vi "Init Menu.vi"(8 "Error In":errorcluster, 9 "Used Items":bool[](array[boolean]), 10 "Item Names":string[][](array[string]), 11 "Menu in":refnum<k9>) -> (0 "Error Out":errorcluster, 3 "menu reference out":refnum<k9>)   [LabVIEW 2019]
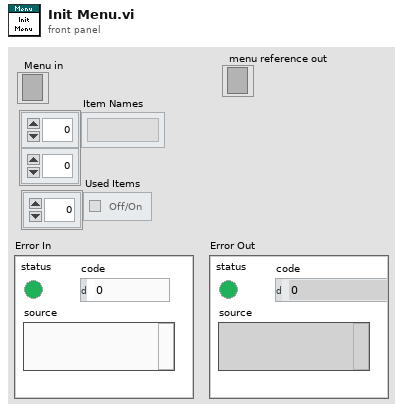
[diagram p1: front panel]
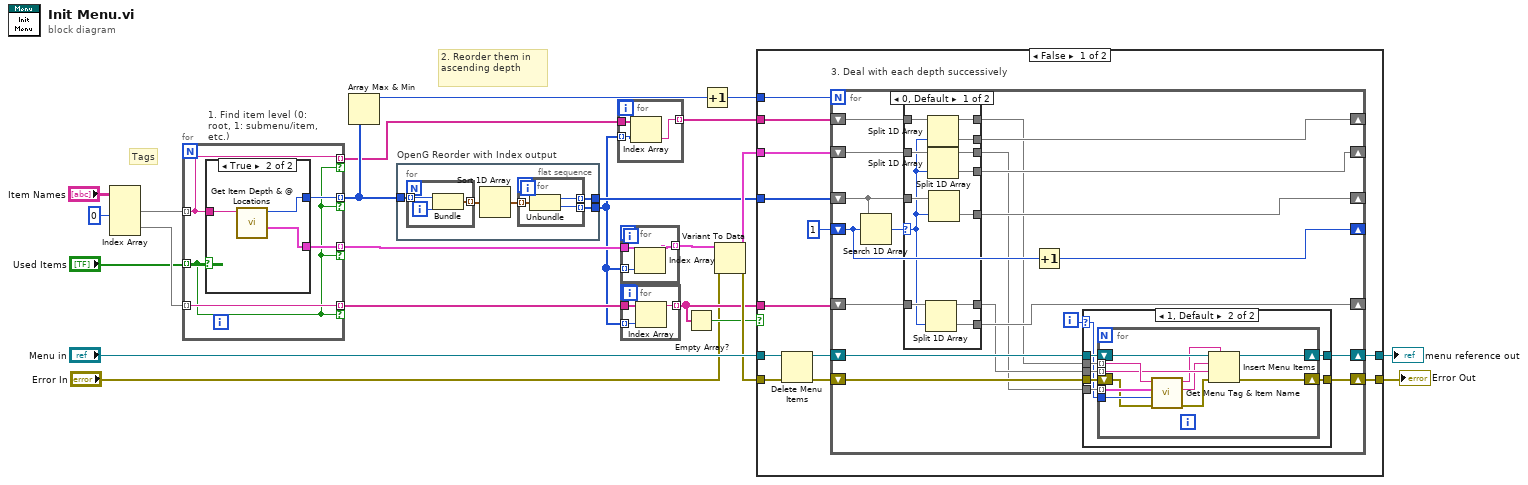
[diagram p0: block diagram]
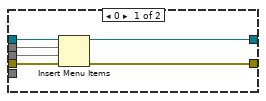
[diagram p3: hidden frame]
diagram:
  # "Tags"
  # "2. Reorder them in ascending depth"
  n1 = Index Array(array="Item Names", index (col) #1=0 ("disabled index (col)")) -> (element #1=w10:string[], element #2=w12:string[])  [unwired: 3 in]
  n2 = for "1. Find item level (0: root, 1: submenu/item, etc.)" {
    tunnel: w10 -> [w25] mode=indexing
    tunnel: [w28] -> w18 mode=indexing if=w24
    tunnel: [w27] -> w21 mode=indexing if=w24
    tunnel: "Used Items" -> [w24] mode=indexing
    tunnel: w12 -> [w26] mode=indexing
    tunnel: [w26] -> w11 mode=indexing if=w24
    tunnel: [w25] -> w1 mode=indexing if=w24
    n3 = case shown="True" w24 {
      tunnel: w25 -> [_ w31]
      tunnel: [_ w29] -> w28
      tunnel: [_ w30] -> w27
      frame False {
      }
      frame True {
        n4 = call "Get Item Depth & @ Locations.vi"("Menu Item Description"=w31) -> ("@ Locations"=w29:cluster{"Array":i32[]}, "Depth"=w30:i32)  [unwired: 8 in, 1 out]
      }
    }
  }
  n5 = Array Max & Min(array=w21) -> (max value=w20:i32)  [unwired: 3 out]
  n6 = flat-sequence "OpenG Reorder with Index output" {
    tunnel: w21 -> [w36]
    tunnel: [w35] -> w14
    tunnel: [w34] -> w3
    frame #0 {
      n7 = for {
        tunnel: w36 -> [w39] mode=indexing
        tunnel: [w37] -> w33 mode=indexing
        i -> [w38]
        n8 = Bundle("Depth"=w39, w38) -> (w37:cluster{"Depth":i32, i32})  [unwired: 1 in]
      }
      n9 = Sort 1D Array(array=w33) -> (sorted array=w32:cluster{"Depth":i32, i32}[])
      n10 = for {
        tunnel: w32 -> [w42] mode=indexing
        tunnel: [w40] -> w35 mode=indexing
        tunnel: [w41] -> w34 mode=indexing
        n11 = Unbundle(w42) -> ("Depth"=w40:i32, w41:i32)
      }
    }
  }
  n12 = for {
    tunnel: w1 -> [w45]
    tunnel: [w44] -> w16 mode=indexing
    tunnel: w3 -> [w43] mode=indexing
    n13 = Index Array(array=w45, index=w43) -> (element=w44:string)
  }
  n14 = for {
    tunnel: w18 -> [w48]
    tunnel: [w47] -> w19 mode=indexing
    tunnel: w3 -> [w46] mode=indexing
    n15 = Index Array(array=w48, index=w46) -> (element=w47:cluster{"Array":i32[]})
  }
  n16 = for {
    tunnel: w11 -> [w51]
    tunnel: [w50] -> w6 mode=indexing
    tunnel: w3 -> [w49] mode=indexing
    n17 = Index Array(array=w51, index=w49) -> (element=w50:string)
  }
  n18 = Empty Array?(array=w6) -> (empty?=w5:bool)
  n19 = Increment(x=w20) -> (x+1=w13:i32)
  n20 = Variant To Data(error in="Error In", type=w18, Variant=w19) -> (data=w17:cluster{"Array":i32[]}[], error out=w7:errorcluster)
  n21 = case shown="False" w5 {
    tunnel: "Menu in" -> [w63 w123]
    tunnel: w17 -> [w61 _]
    tunnel: w16 -> [w59 _]
    tunnel: [w58 w124] -> w15
    tunnel: w14 -> [w57 _]
    tunnel: w13 -> [w56 _]
    tunnel: w7 -> [w55 w124]
    tunnel: w6 -> [w53 _]
    tunnel: [w52 w123] -> w2
    frame False {
      n22 = Delete Menu Items(6:w55, 9:w63) -> (0:w54:errorcluster, 3:w60:refnum<k9>)  [unwired: 2 in]
      n23 = for "3. Deal with each depth successively" {
        N: w56 -> [_]
        shift-right: [w81] -> _
        shift-left: w57 -> [w82]
        shift-right: [w79] -> _
        shift-left: 1 ("max value") -> [w80]
        shift-right: [w77] -> _
        shift-left: w61 -> [w78]
        shift-right: [w75] -> _
        shift-left: w53 -> [w76]
        shift-right: [w73] -> w52
        shift-left: w60 -> [w74]
        shift-right: [w71] -> w58
        shift-left: w54 -> [w72]
        shift-right: [w67] -> _
        shift-left: w59 -> [w69]
        i -> [w65]
        n24 = Search 1D Array(1D array=w82, element=w80) -> (index of element=w68:i32)  [unwired: 1 in]
        n25 = case shown="0, Default" w68 {
          selector: w68 -> [w83 _]
          tunnel: w82 -> [w94 _]
          tunnel: [w93 _] -> w81
          tunnel: w78 -> [w92 w96]
          tunnel: [w91 _] -> w77
          tunnel: w76 -> [w90 w95]
          tunnel: [w89 _] -> w75
          tunnel: [w88 w95] -> w70
          tunnel: w69 -> [w87 w97]
          tunnel: [w86 _] -> w67
          tunnel: [w85 w97] -> w66
          tunnel: [w84 w96] -> w64
          frame 0, Default {
            n26 = Split 1D Array(array=w90, index=w83) -> (first subarray=w88:string[], second subarray=w89:string[])
            n27 = Split 1D Array(array=w87, index=w83) -> (first subarray=w85:string[], second subarray=w86:string[])
            n28 = Split 1D Array(array=w92, index=w83) -> (first subarray=w84:cluster{"Array":i32[]}[], second subarray=w91:cluster{"Array":i32[]}[])
            n29 = Split 1D Array(array=w94, index=w83) -> (second subarray=w93:i32[])  [unwired: 1 out]
          }
          frame -1 {
          }
        }
        n30 = Increment(x=w80) -> (x+1=w79:i32)
        n31 = case shown="1, Default" w65 {
          selector: w65 -> [_ w104]
          tunnel: w74 -> [w103 w111]
          tunnel: [w102 w110] -> w73
          tunnel: w72 -> [w101 w109]
          tunnel: [w99 w108] -> w71
          tunnel: w70 -> [w100 w106]
          tunnel: w66 -> [w98 w107]
          tunnel: w64 -> [_ w105]
          frame 0 {
            n32 = Insert Menu Items(6:w101, 7:w100, 8:w98, 9:w103) -> (0:w99:errorcluster, 3:w102:refnum<k9>)  [unwired: 2 in, 1 out]
          }
          frame 1, Default {
            n33 = for {
              shift-right: [w121] -> w110
              shift-left: w111 -> [w122]
              shift-right: [w114] -> w108
              shift-left: w109 -> [w116]
              tunnel: w107 -> [w120] mode=indexing
              tunnel: w106 -> [w119] mode=indexing
              tunnel: w105 -> [w118] mode=indexing
              tunnel: w104 -> [w117]
              n34 = call "Get Menu Tag & Item Name.vi"("error in (no error)"=w116, "Item Depth"=w117, "@ Locations"=w118, "Menu Item Description"=w120) -> ("error out"=w115:errorcluster, "Item Name"=w112:string, "Menu Tag"=w113:string)  [unwired: 5 in]
              n35 = Insert Menu Items(5:w113, 6:w115, 7:w119, 8:w112, 9:w122) -> (0:w114:errorcluster, 3:w121:refnum<k9>)  [unwired: 1 in, 1 out]
            }
          }
        }
      }
    }
    frame True {
    }
  }
  "Error Out" <- w15
  "menu reference out" <- w2
